vi "Status Size.vi"(8 "error in (no error)":errorcluster) -> (0 "error out":errorcluster, 3 "size":u64 format="%d bytes")   [LabVIEW 2017, in "DSF Core.lvlib" / "Status Pointer.lvclass"]
uses:
  Status Pointer.lvclass
  Status Data.ctl
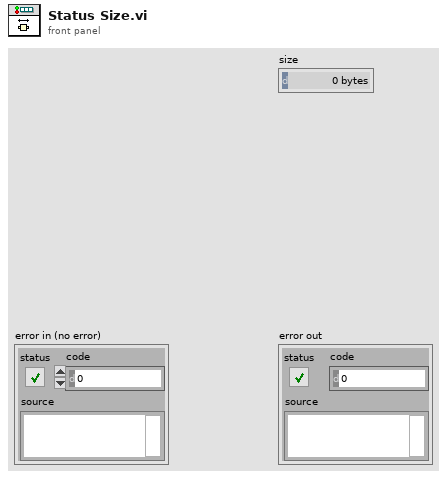
[diagram p1: front panel]
types:
  T1 = typedef "DSF Core.lvlib/Status Pointer.lvclass/Status Data.ctl" = cluster{"late count":u64, "iteration":u64, "rx duration":u32, "tx duration":u32}
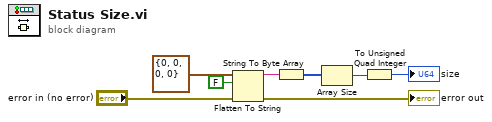
[diagram p0: block diagram]
diagram:
  n1 = Flatten To String(anything=T1 {"late count"=0, "iteration"=0, "rx duration"=0, "tx duration"=0} ("Transfer Group status"), prepend array or string size? (T)=FALSE, error in (no error)="error in (no error)") -> (data string=w7:string, error out=→"error out":errorcluster)  [unwired: 1 in, 1 out]
  n2 = String To Byte Array(string=w7) -> (unsigned byte array=w6:u8[])
  n3 = Array Size(array=w6) -> (size(s)=w5:i32)
  n4 = To Unsigned Quad Integer(1:w5) -> (0:→"size":u64)
